vi "Stop Stream and Reset RX FIFO.vi"(8 "error in (no error)":errorcluster, 10 "2 USRPs?":bool[](array[boolean]), 11 "Refnum in":refnum<k20>[](array[refnum])) -> (0 "error out":errorcluster, 3 "Refnum out":refnum<k20>[](array[refnum]))   [LabVIEW 2016]
uses:
  <instrlib>/_niInstr/Streaming/v1/Host/niInstr Streaming v1 Host.lvlib
  6592R/SubVIs/Aurora Stream (NI 6592R) (Host).lvlib
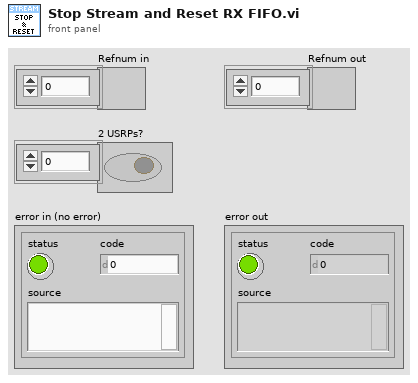
[diagram p1: front panel]
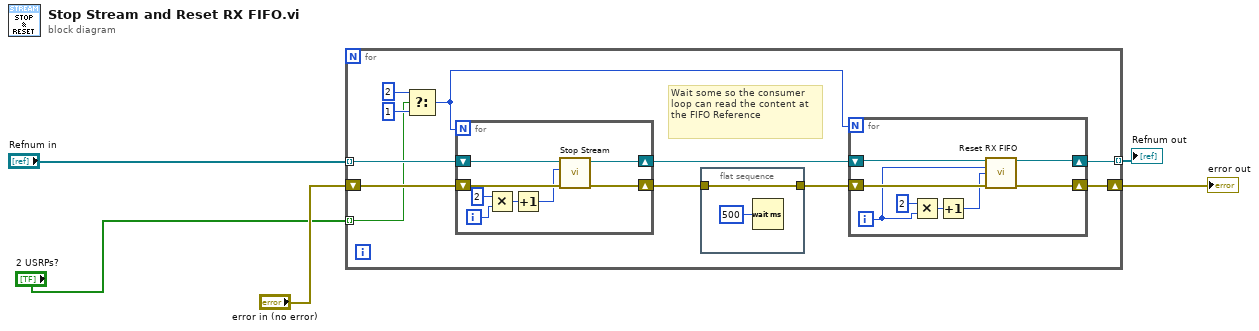
[diagram p0: block diagram]
diagram:
  n1 = for {
    tunnel: "Refnum in" -> [w15] mode=indexing
    tunnel: [w9] -> w2 mode=indexing
    shift-right: [w10] -> w3
    shift-left: "error in (no error)" -> [w16]
    tunnel: "2 USRPs?" -> [w12] mode=indexing
    # "Wait some so the consumer loop can read the content at the FIFO Reference"
    n2 = Select(t=2, s=w12, f=1) -> (s? t:f=w6:i32)
    n3 = for {
      N: w6 -> [_]
      shift-right: [w32] -> w11
      shift-left: w15 -> [w33]
      shift-right: [w31] -> w8
      shift-left: w16 -> [w34]
      i -> [w28]
      n4 = Multiply(x=2, y=w28) -> (x*y=w29:i32)
      n5 = Increment(x=w29) -> (x+1=w27:i32)
      n6 = call <instrlib>:"Stop Stream.vi"("error in (no error)"=w34, "stream index"=w27, "refnum in"=w33) -> ("error out"=w31:errorcluster, "refnum out"=w32:refnum<k20>)  [unwired: 5 in, 2 out]
    }
    n7 = flat-sequence {
      tunnel: w8 -> [w18]
      tunnel: [w18] -> w7
      frame #0 {
        n8 = Wait (ms)(milliseconds to wait=u32 500) -> ()  [unwired: 1 out]
      }
    }
    n9 = for {
      N: w6 -> [_]
      shift-right: [w24] -> w9
      shift-left: w11 -> [w25]
      shift-right: [w23] -> w10
      shift-left: w7 -> [w26]
      i -> [w20]
      n10 = Multiply(x=2, y=w20) -> (x*y=w22:i32)
      n11 = Increment(x=w22) -> (x+1=w19:i32)
      n12 = call "Reset RX FIFO.vi"("Refnum in"=w25, "Port"=w20, "stream index"=w19, "error in"=w26) -> ("Refnum out"=w24:refnum<k20>, "error out"=w23:errorcluster)  [unwired: 10 in]
    }
  }
  "error out" <- w3
  "Refnum out" <- w2
